vi "Item Modify.vi"(0 "Tree Reference In":refnum<vi>, 1 "Tag to Modify (Current)":string, 2 "New Tag Value (No Change)":string, 3 "New Text Value":string, 5 "error in (no error)":errorcluster, 7 "Symbol(-1:No Change)":i32=-1, 9 "Column # (0)":i32) -> (14 "Tree Reference Out":refnum<vi>, 19 "error out":errorcluster)   [LabVIEW 2011, in "VITesterUtilities.lvlib"]
doc: "Modifies an item in the tree. Uses the current item if input is blank. Allows to modify both the tag and text"
uses:
  Libraries/VITesterUtilities.lvlib
panel:
  # "VI INPUTS"
  # "VI OUTPUTS"
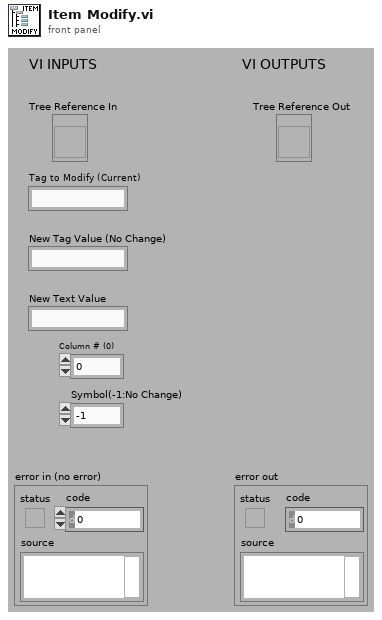
[diagram p1: front panel]
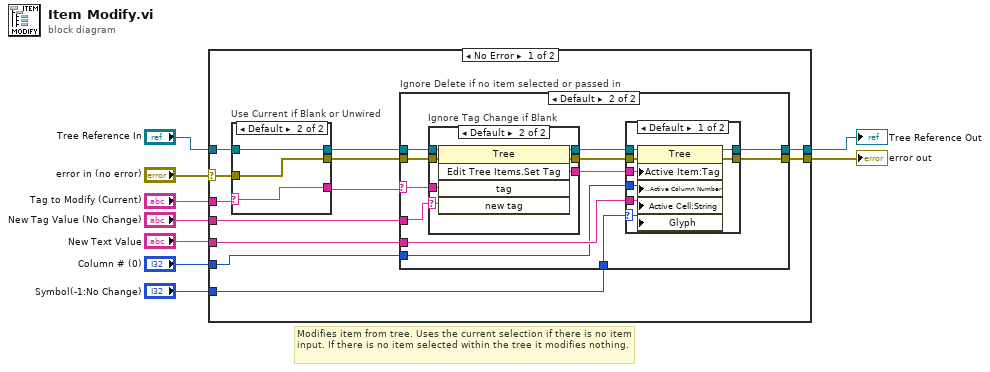
[diagram p0: block diagram]
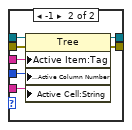
[diagram p3: hidden frame]
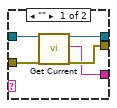
[diagram p5: hidden frame]
diagram:
  # "Modifies item from tree. Uses the current selection if there is no item input. If there is no item selected within the tree it modifies nothing."
  n1 = case shown="No Error" "error in (no error)" {
    selector: "error in (no error)" -> [w19 w69]
    tunnel: "Tree Reference In" -> [w21 w70]
    tunnel: [w18 w70] -> w8
    tunnel: [w17 w69] -> w7
    tunnel: "Tag to Modify (Current)" -> [w20 _]
    tunnel: "New Text Value" -> [w13 _]
    tunnel: "New Tag Value (No Change)" -> [w12 _]
    tunnel: "Column # (0)" -> [w11 _]
    tunnel: "Symbol(-1:No Change)" -> [w10 _]
    frame No Error {
      n2 = case "Use Current if Blank or Unwired" shown="Default" w20 {
        selector: w20 -> [_ w66]
        tunnel: [w64 w68] -> w16
        tunnel: w21 -> [w65 w68]
        tunnel: [w63 w67] -> w15
        tunnel: w19 -> [w62 w67]
        tunnel: [w61 w66] -> w14
        frame "" {
          n3 = call "Get Current.vi"("Tree Reference In"=w65, "error in (no error)"=w62) -> ("Tree Reference Out"=w64:refnum<vi>, "Current Tag"=w61:string, "error out"=w63:errorcluster)  [unwired: 14 in, 1 out]
        }
        frame Default {
        }
      }
      n4 = case "Ignore Delete if no item selected or passed in" shown="Default" w14 {
        selector: w14 -> [_ w30]
        tunnel: [w23 w32] -> w18
        tunnel: [w22 w31] -> w17
        tunnel: w16 -> [w23 w33]
        tunnel: w15 -> [w22 w35]
        tunnel: w13 -> [_ w28]
        tunnel: w12 -> [_ w26]
        tunnel: w11 -> [_ w25]
        tunnel: w10 -> [_ w24]
        frame "" {
        }
        frame Default {
          n5 = case "Ignore Tag Change if Blank" shown="Default" w26 {
            selector: w26 -> [_ w54]
            tunnel: w35 -> [w52 w60]
            tunnel: [w52 w59] -> w34
            tunnel: w33 -> [w53 w58]
            tunnel: w30 -> [w51 w57]
            tunnel: [w51 w56] -> w29
            tunnel: [w53 w55] -> w27
            frame "" {
            }
            frame Default {
              n6 = invoke class="Tree" method="Edit Tree Items.Set Tag"(reference=w58, error in=w60, "tag"=w57, "new tag"=w54) -> (reference out=w55:refnum<vi>, error out=w59:errorcluster, "Edit Tree Items:Set Tag"=w56:string)  [unwired: 1 in, 2 out]
            }
          }
          n7 = case shown="Default" w24 {
            selector: w24 -> [w36 _]
            tunnel: w34 -> [w43 w50]
            tunnel: [w42 w49] -> w32
            tunnel: [w41 w48] -> w31
            tunnel: w29 -> [w40 w47]
            tunnel: w28 -> [w39 w46]
            tunnel: w27 -> [w38 w45]
            tunnel: w25 -> [w37 w44]
            frame Default {
              n8 = property class="Tree"(reference=w38, error in=w43, "Active Item:Tag"=w40, "Active Cell:Active Column Number"=w37, "Active Cell:String"=w39, "Glyph"=w36) -> (reference out=w42:refnum<vi>, error out=w41:errorcluster)
            }
            frame -1 {
              n9 = property class="Tree"(reference=w45, error in=w50, "Active Item:Tag"=w47, "Active Cell:Active Column Number"=w44, "Active Cell:String"=w46) -> (reference out=w49:refnum<vi>, error out=w48:errorcluster)
            }
          }
        }
      }
    }
    frame Error {
    }
  }
  "Tree Reference Out" <- w8
  "error out" <- w7
